vi "config filepaths.vi"(8 "error in (no error)":errorcluster) -> (0 "error out":errorcluster, 4 "Methods":string[](array[string]))   [LabVIEW 2012]
uses:
  Folders.ctl
  Paths.ctl
  SVN.ctl
  Mail Server.ctl
  ReadWrite.ctl
  ADT 2/AguaClara Library.lvlib
  Design Server.lvlib
panel:
  out "valid email":bool
  out "Mail Server in":T1={"Outgoing Mail Server (SMTP)"="smtp.gmail.com", "MAIL Account User ID"="monroews", "MAIL Account Password"="", "Enable SSL"=TRUE, "Port"=587, "Sender's Email Address"="monroews@gmail.com", "Sender's Name"="Monroe Weber-Shirk"}
  in  "Mail Server":T1={"Outgoing Mail Server (SMTP)"="smtp.gmail.com", "MAIL Account User ID"="monroews", "MAIL Account Password"="", "Enable SSL"=TRUE, "Port"=587, "Sender's Email Address"="monroews@gmail.com", "Sender's Name"="Monroe Weber-Shirk"}
  out "Paths in":T2
  out "SVN in":T3
  out "Paths ok":bool
  out "SVN ok":bool
  in  "Abort":bool
  in  "SVN":T3
  in  "Paths":T2
  in  "Cancel Button":bool
  in  "OK Button":bool
  in  "Folders":T4
  # "https://forge.cornell.edu/svn/repos/automated_design/Final Designs/"
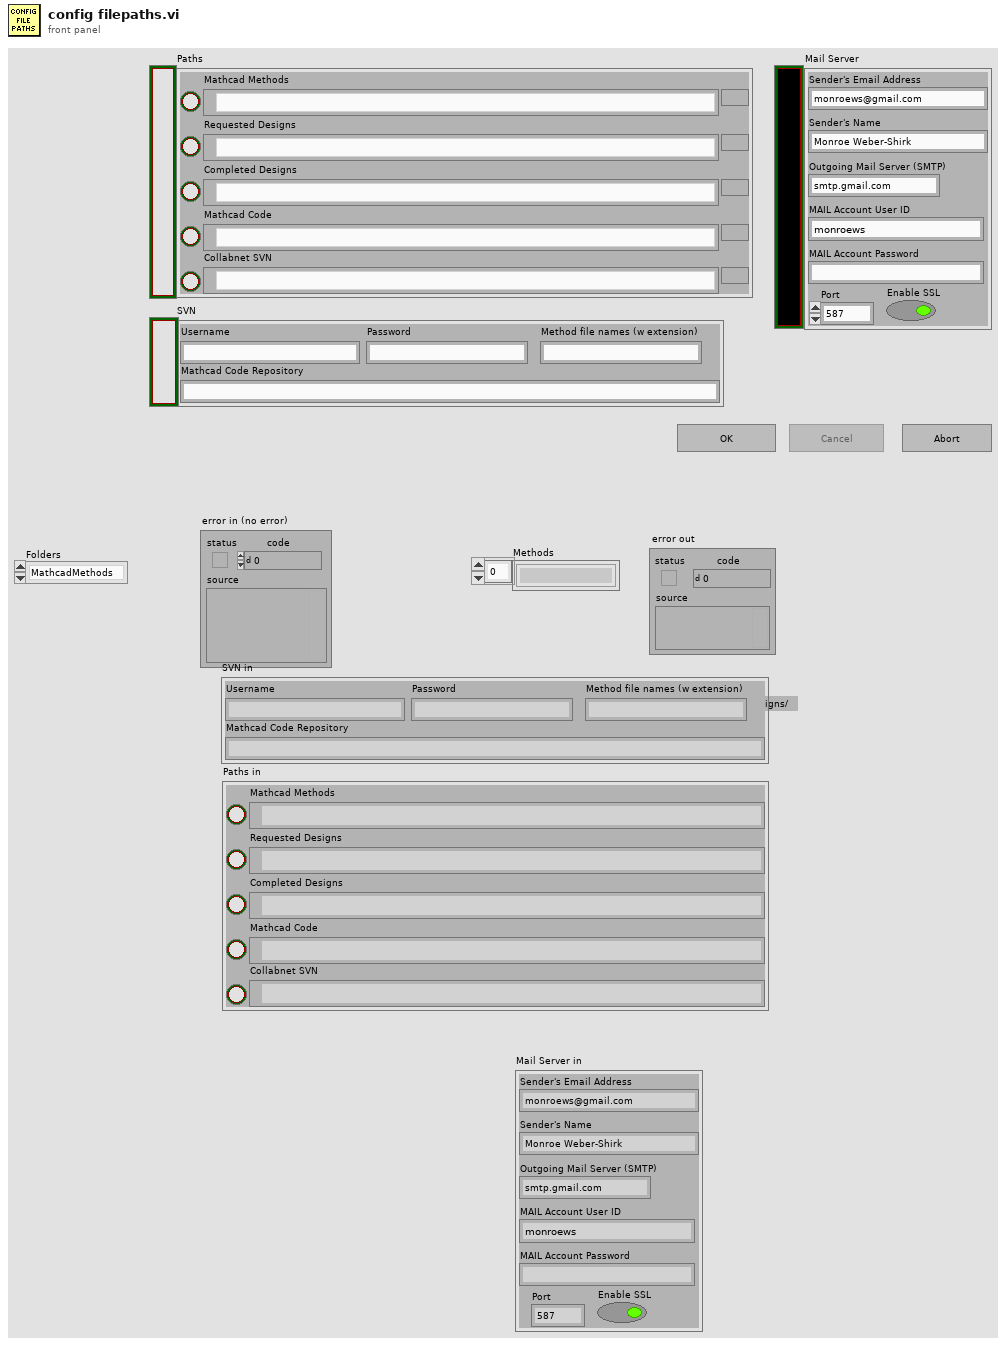
[diagram p1: front panel]
types:
  T1 = typedef "Mail Server.ctl" = cluster{"Outgoing Mail Server (SMTP)":string, "MAIL Account User ID":string, "MAIL Account Password":string, "Enable SSL":bool, "Port":i32, "Sender's Email Address":string, "Sender's Name":string}
  T2 = typedef "Paths.ctl" = cluster{"Mathcad Methods":path, "Requested Designs":path, "Completed Designs":path, "Mathcad Code":path, "Collabnet SVN":path, "Mathcad Methods ok":bool, "Requested Designs ok":bool, "Completed Designs ok":bool, "Mathcad Code ok":bool, "Collabnet SVN":bool}
  T3 = typedef "SVN.ctl" = cluster{"Mathcad Code Repository":string, "Username":string, "Password":string, "Method file names (w extension)":string}
  T4 = typedef "Design Server.lvlib/Folders.ctl" = enum16{"MathcadMethods", "RequestedDesigns", "CompletedDesigns", "MathcadCode", "CollabnetSVN.exe"}
  T5 = enum8{"Enabled", "Disabled", "Disabled and Grayed Out"}
  T6 = typedef "ReadWrite.ctl" = enum16{"Read", "Write"}
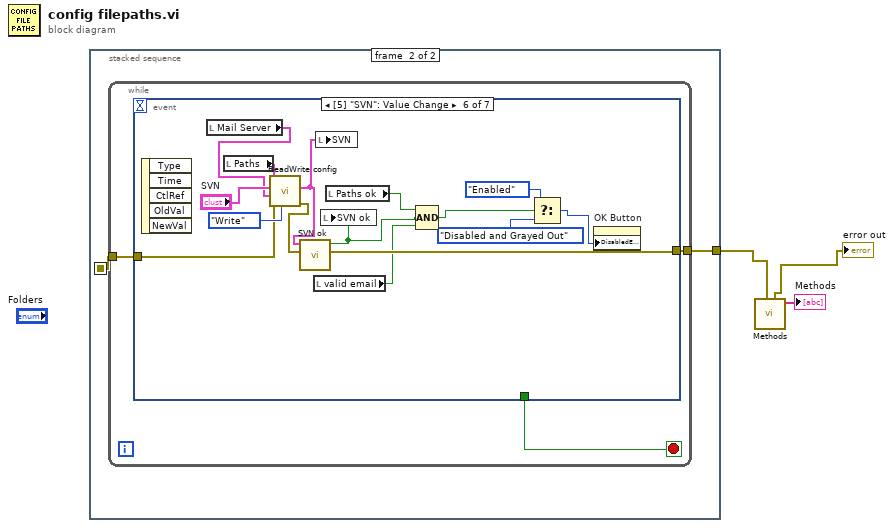
[diagram p0: block diagram]
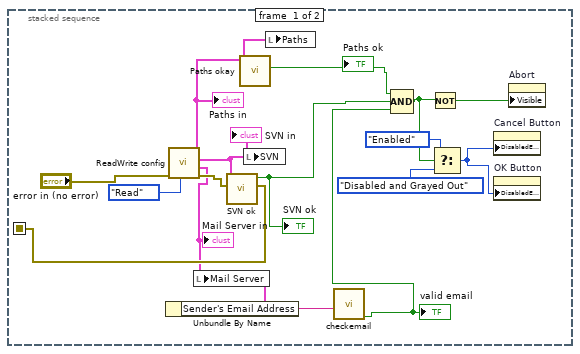
[diagram p2: hidden frame]
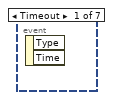
[diagram p3: hidden frame]
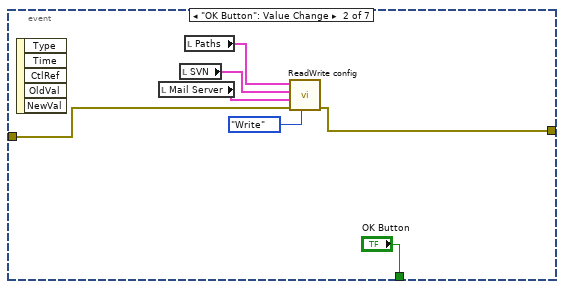
[diagram p4: hidden frame]
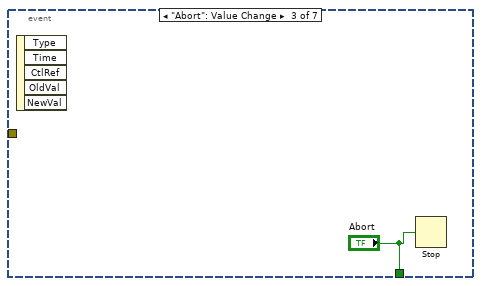
[diagram p5: hidden frame]
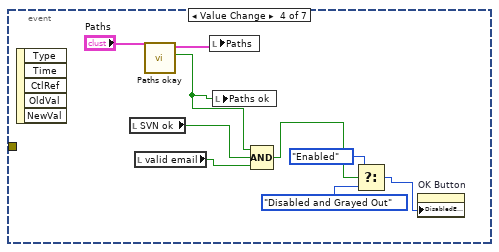
[diagram p6: hidden frame]
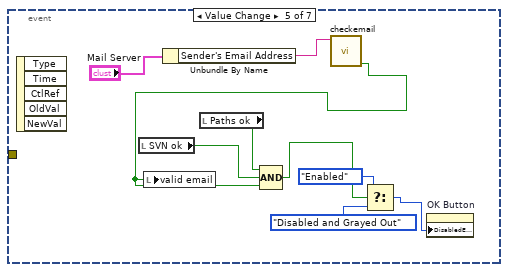
[diagram p7: hidden frame]
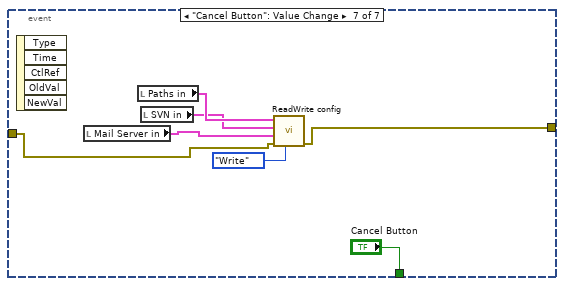
[diagram p8: hidden frame]
diagram:
  n1 = stacked-sequence {
    seq-local: [w14 _] -> [_ w21]
    tunnel: [_ w22] -> w2
    frame #0 {
      n2 = call "ReadWrite config.vi"("Config"=ReadWrite."Read", "error in (no error)"="error in (no error)") -> ("error out"=w15:errorcluster, "Mail Server"=w9:T1, "SVN"=w16:T3, "Paths"=w18:T2)  [unwired: 6 in]
      "SVN in" <- w16
      "Paths in" <- w18
      "Mail Server in" <- w9
      n3 = Unbundle By Name(w9) -> ("Sender's Email Address"=w8:string)
      n4 = local write "Mail Server"(w9) -> ()
      n5 = call "SVN ok.vi"("error in"=w15, "SVN in"=w16) -> ("error out"=w14:errorcluster, "SVN ok"=w6:bool)  [unwired: 8 in]
      "SVN ok" <- w6
      n6 = call "Paths okay.vi"("Paths"=w18) -> ("passed"=w7:bool, "Paths out"=w17:T2)  [unwired: 9 in]
      "Paths ok" <- w7
      n7 = local write "SVN"(w16) -> ()
      n8 = local write "Paths"(w17) -> ()
      n9 = call "checkemail.vi"("email"=w8) -> ("valid email"=w4:bool)  [unwired: 7 in, 3 out]
      "valid email" <- w4
      n10 = Compound Arithmetic op=AND(w7, w6, w4) -> (w5:bool)
      n11 = Not(x=w5) -> (.not. x?=w13:bool)
      n12 = Select(t=T5."Enabled" ("Disabled"), s=w5, f=T5."Disabled and Grayed Out" ("Disabled")) -> (s? t:f=w10:T5)
      n13 = property on="Cancel Button" class="Bool"("DisabledEnum"=w10) -> ()  [unwired: 2 in, 2 out]
      n14 = property on="OK Button" class="Bool"("DisabledEnum"=w10) -> ()  [unwired: 2 in, 2 out]
      n15 = property on="Abort" class="Bool"("Visible"=w13) -> ()  [unwired: 2 in, 2 out]
    }
    frame #1 {
      n16 = while {
        tunnel: w21 -> [w24]
        tunnel: [w23] -> w22
        stop <- w25 stop-if-true
        n17 = event shown="[5] \"SVN\": Value Change" {
          selector: _ -> [_ _ _ _ _ _ _]
          dyn-events: _ -> [_ _ _ _ _ _ _]
          timeout: _ -> [_ _ _ _ _ _ _]
          tunnel: [_ "OK Button" "Abort" _ _ _ "Cancel Button"] -> w25
          tunnel: w24 -> [_ w28 _ _ _ w59 w69]
          tunnel: [_ w27 _ _ _ w66 w68] -> w23
          event Timeout {
            n18 = event-data() -> ()  [unwired: 1 in, 2 out]
          }
          event "OK Button": Value Change {
            n19 = event-data() -> ()  [unwired: 1 in, 5 out]
            n20 = local read "Mail Server"() -> (w26:T1)
            n21 = local read "SVN"() -> (w31:T3)
            n22 = local read "Paths"() -> (w30:T2)
            n23 = call "ReadWrite config.vi"("Config"=ReadWrite."Write", "error in (no error)"=w28, "Mail Server in"=w26, "SVN in"=w31, "Paths in"=w30) -> ("error out"=w27:errorcluster)  [unwired: 3 in, 3 out]
          }
          event "Abort": Value Change {
            n24 = event-data() -> ()  [unwired: 1 in, 5 out]
            n25 = Stop(stop? (T)="Abort") -> ()
          }
          event Value Change {
            n26 = event-data() -> ()  [unwired: 1 in, 5 out]
            n27 = local read "SVN ok"() -> (w36:bool)
            n28 = local read "valid email"() -> (w37:bool)
            n29 = call "Paths okay.vi"("Paths"="Paths") -> ("passed"=w35:bool, "Paths out"=w41:T2)  [unwired: 9 in]
            n30 = local write "Paths"(w41) -> ()
            n31 = local write "Paths ok"(w35) -> ()
            n32 = Compound Arithmetic op=AND(w35, w36, w37) -> (w34:bool)
            n33 = Select(t=T5."Enabled" ("Disabled"), s=w34, f=T5."Disabled and Grayed Out" ("Disabled")) -> (s? t:f=w38:T5)
            n34 = property on="OK Button" class="Bool"("DisabledEnum"=w38) -> ()  [unwired: 2 in, 2 out]
          }
          event Value Change {
            n35 = event-data() -> ()  [unwired: 1 in, 5 out]
            n36 = local read "SVN ok"() -> (w48:bool)
            n37 = Unbundle By Name("Mail Server") -> ("Sender's Email Address"=w44:string)
            n38 = local read "Paths ok"() -> (w47:bool)
            n39 = call "checkemail.vi"("email"=w44) -> ("valid email"=w43:bool)  [unwired: 7 in, 3 out]
            n40 = local write "valid email"(w43) -> ()
            n41 = Compound Arithmetic op=AND(w47, w48, w43) -> (w46:bool)
            n42 = Select(t=T5."Enabled" ("Disabled"), s=w46, f=T5."Disabled and Grayed Out" ("Disabled")) -> (s? t:f=w49:T5)
            n43 = property on="OK Button" class="Bool"("DisabledEnum"=w49) -> ()  [unwired: 2 in, 2 out]
          }
          event Value Change {
            n44 = event-data() -> ()  [unwired: 1 in, 5 out]
            n45 = local read "Mail Server"() -> (w52:T1)
            n46 = local read "Paths"() -> (w61:T2)
            n47 = call "ReadWrite config.vi"("Config"=ReadWrite."Write", "error in (no error)"=w59, "Mail Server in"=w52, "SVN in"="SVN", "Paths in"=w61) -> ("error out"=w58:errorcluster, "SVN"=w53:T3)  [unwired: 3 in, 2 out]
            n48 = call "SVN ok.vi"("error in"=w58, "SVN in"=w53) -> ("error out"=w66:errorcluster, "SVN ok"=w56:bool)  [unwired: 8 in]
            n49 = local read "valid email"() -> (w57:bool)
            n50 = local write "SVN"(w53) -> ()
            n51 = local write "SVN ok"(w56) -> ()
            n52 = local read "Paths ok"() -> (w55:bool)
            n53 = Compound Arithmetic op=AND(w55, w56, w57) -> (w54:bool)
            n54 = Select(t=T5."Enabled" ("Disabled"), s=w54, f=T5."Disabled and Grayed Out" ("Disabled")) -> (s? t:f=w63:T5)
            n55 = property on="OK Button" class="Bool"("DisabledEnum"=w63) -> ()  [unwired: 2 in, 2 out]
          }
          event "Cancel Button": Value Change {
            n56 = event-data() -> ()  [unwired: 1 in, 5 out]
            n57 = local read "Mail Server in"() -> (w67:T1)
            n58 = local read "Paths in"() -> (w71:T2)
            n59 = local read "SVN in"() -> (w70:T3)
            n60 = call "ReadWrite config.vi"("Config"=ReadWrite."Write", "error in (no error)"=w69, "Mail Server in"=w67, "SVN in"=w70, "Paths in"=w71) -> ("error out"=w68:errorcluster)  [unwired: 3 in, 3 out]
          }
        }
      }
    }
  }
  n61 = call "Methods.vi"("error in"=w2) -> ("Methods"=→"Methods":string[], "error out"=→"error out":errorcluster)  [unwired: 9 in]
